vi "Dereference Bitmap.vi"(5 "Back":u32(colorbox)=16448250, 6 "Alpha":u8=255, 7 "Front":u32(colorbox), 8 "error in (no error)":errorcluster, 11 "bitmap":T2) -> (0 "error out":errorcluster, 3 "image data":T1)   [LabVIEW 2023, in "Freetype Drawer.lvlib"]
uses:
  Freetype Drawer.lvlib
  FT Bitmap.ctl
  <vilib>/picture/picture.llb/imagedata.ctl
  Font Glyph Drawer Interface/Font Glyph Drawer Interface.lvlib
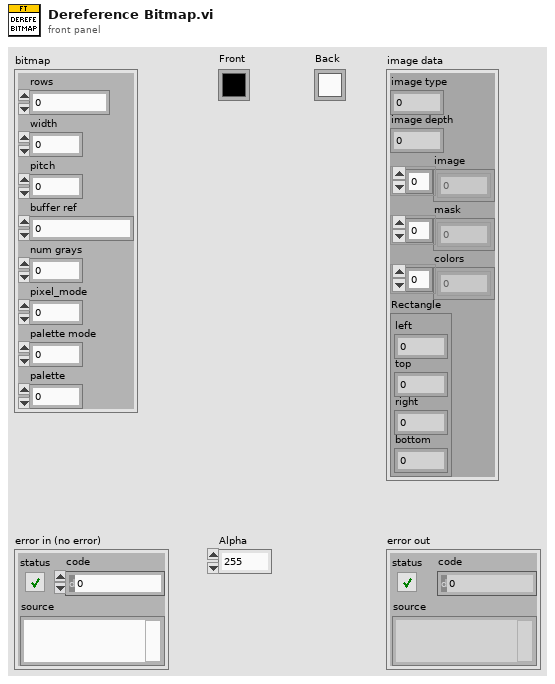
[diagram p1: front panel]
types:
  T1 = typedef "imagedata.ctl" = cluster{"image type":i32, "image depth":i32, "image":u8[], "mask":u8[], "colors":u32[], "Rectangle":cluster{"left":i16, "top":i16, "right":i16, "bottom":i16}}
  T2 = typedef "Freetype Drawer.lvlib/FT Bitmap.ctl" = cluster{"rows":u32, "width":u32, "pitch":i32, "buffer ref":i64, "num grays":i16, "pixel_mode":u8, "palette mode":u8, "palette":i64}
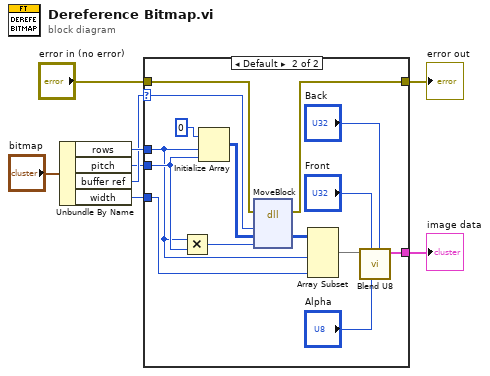
[diagram p0: block diagram]
diagram:
  n1 = Unbundle By Name("bitmap") -> ("rows"=w5:u32, "pitch"=w3:i32, "buffer ref"=w4:i64, "width"=w1:u32)
  n2 = case shown="Default" w4 {
    selector: w4 -> [_ w22]
    tunnel: [w9 w24] -> w8
    tunnel: "error in (no error)" -> [w9 w23]
    tunnel: w5 -> [_ w11]
    tunnel: w3 -> [_ w20]
    tunnel: [_ w17] -> w2
    tunnel: w1 -> [_ w12]
    frame 0 {
    }
    frame Default {
      n3 = Multiply(x=w11, y=w20) -> (x*y=w19:u32)
      n4 = Initialize Array(u8 0 ("Numeric"), w11, w20) -> (w21:u8[][])
      n5 = dll-call lib="LabVIEW" fn="MoveBlock"(error in=w23, "in"=w22, "out"=w21, "size"=w19) -> (error out=w24:errorcluster, "out"=w18:u8[][])  [unwired: 5 in, 1 out]
      n6 = Array Subset(array=w18, length (row)=w11, length (col)=w12) -> (w14:u8[][])  [unwired: 2 in]
      n7 = call "Blend U8.vi"("Back"="Back", "Alpha"="Alpha", "Front"="Front", "U8"=w14) -> ("image data"=w17:T1)  [unwired: 7 in]
    }
  }
  "error out" <- w8
  "image data" <- w2
